vi "Tree Interaction.vi"() -> ()   [LabVIEW 2020, in "NI_VIAnCFGDataStructure.lvlib" / "Tree.lvclass"]
uses:
  <vilib>/addons/analyzer/VIAnCFGDataStructure/Tree Manager/Tree.lvclass
  <vilib>/addons/analyzer/VIAnCFGDataStructure/Tree Manager/API/Set Attribute.vi
  <vilib>/addons/analyzer/VIAnCFGDataStructure/Tree Manager/API/Get Name.vi
  <vilib>/addons/analyzer/VIAnCFGDataStructure/Tree Manager/API/Get Attribute.vi
panel:
  out "Tag":string
  out "Attribute Value":variant
  out "Clicked Attribute Name":string
  out "Clicked Tree Name":string
  in  "Stop Button":bool
  in  "Tree":string(tree)
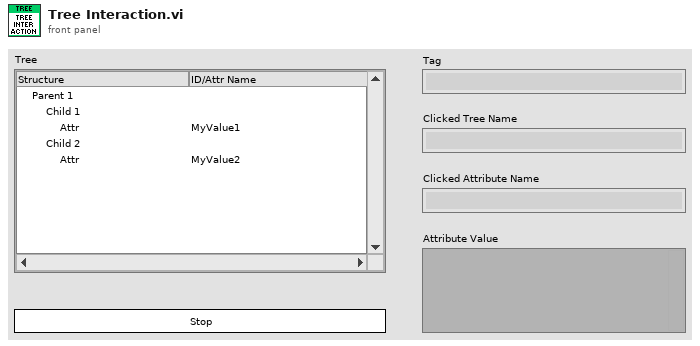
[diagram p1: front panel]
types:
  T1 = typedef "NI_VIAnCFGDataStructure.lvlib/Tree.lvclass/Session Handle.ctl" = refnum<data-value>
  T2 = typedef "LVPoint32TypeDef.ctl" = cluster{"Horizontal":i32, "Vertical":i32}
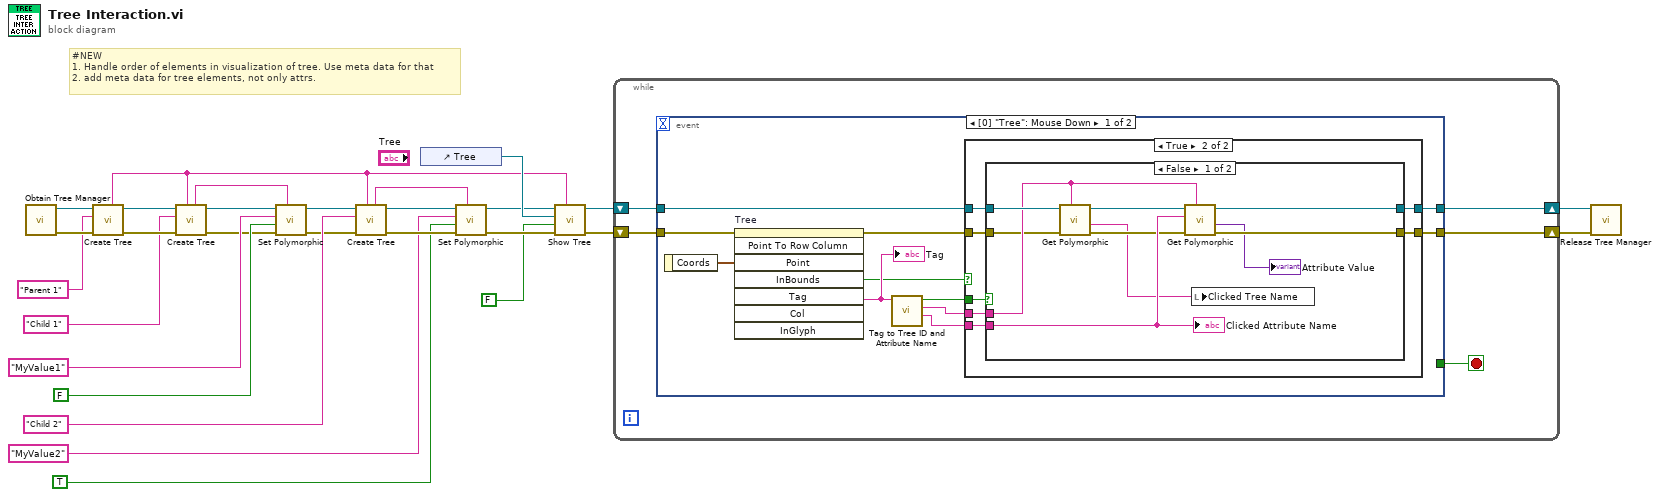
[diagram p0: block diagram]
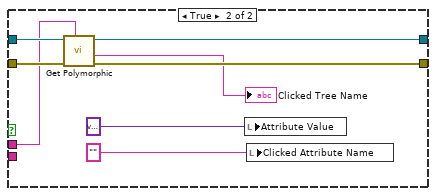
[diagram p3: hidden frame]
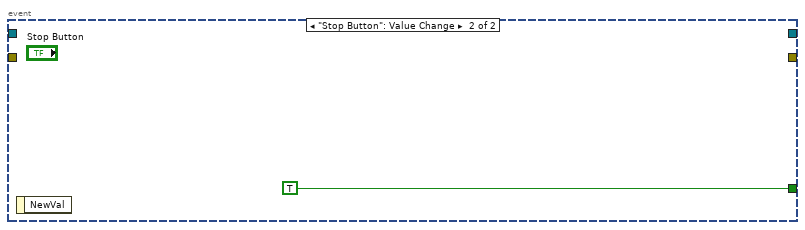
[diagram p4: hidden frame]
diagram:
  # "#NEW\n1. Handle order of elements in visualization of tree. Use meta data for that\n2. add meta data for tree elements, not only attrs."
  n1 = call <vilib>:"Obtain Tree Manager.vi"() -> ("Error Out"=w27:errorcluster, "Tree"=w28:T1)  [unwired: 10 in]
  n2 = call <vilib>:"Create Tree.vi"("Error In"=w27, "Name"="Parent 1", "Tree Manager"=w28) -> ("Error Out"=w25:errorcluster, "Tree Manager"=w26:T1, "Unique ID"=w4:string)  [unwired: 6 in]
  n3 = call <vilib>:"Create Tree.vi"("Parent ID (empty)"=w4, "Error In"=w25, "Name"="Child 1", "Tree Manager"=w26) -> ("Error Out"=w7:errorcluster, "Tree Manager"=w12:T1, "Unique ID"=w3:string)  [unwired: 5 in]
  n4 = call-poly <vilib>:"Set Polymorphic.vi"("Tree ID"=w3, "Error In"=w7, "Attribute Value"=FALSE, "Attribute Name"="MyValue1" ("Name"), "Tree Manager"=w12) -> ("Error Out"=w10:errorcluster, "Tree Manager"=w11:T1)  [unwired: 4 in, 1 out]
  n5 = call <vilib>:"Create Tree.vi"("Parent ID (empty)"=w4, "Error In"=w10, "Name"="Child 2", "Tree Manager"=w11) -> ("Error Out"=w17:errorcluster, "Tree Manager"=w18:T1, "Unique ID"=w2:string)  [unwired: 5 in]
  n6 = control-ref of="Tree"() -> (w21:refnum<vi>)
  n7 = call-poly <vilib>:"Set Polymorphic.vi"("Tree ID"=w2, "Error In"=w17, "Attribute Value"=TRUE, "Attribute Name"="MyValue2" ("Name"), "Tree Manager"=w18) -> ("Error Out"=w13:errorcluster, "Tree Manager"=w14:T1)  [unwired: 4 in, 1 out]
  n8 = call <vilib>:"Show Tree.vi"("Root ID"=w4, "Error In"=w13, "Show IDs (False)"=FALSE ("Show IDs (True)"), "Tree Ref"=w21, "Tree"=w14) -> ("Error Out"=w19:errorcluster, "Tree"=w20:T1)  [unwired: 5 in]
  n9 = while {
    shift-right: [w29] -> w6
    shift-left: w20 -> [w31]
    shift-right: [w30] -> w5
    shift-left: w19 -> [w32]
    stop <- w33 stop-if-true
    n10 = event shown="[0] \"Tree\": Mouse Down" {
      selector: _ -> [_ _]
      dyn-events: _ -> [_ _]
      timeout: _ -> [_ _]
      tunnel: [_ TRUE] -> w33
      tunnel: w32 -> [w42 _]
      tunnel: w31 -> [w38 _]
      tunnel: [w36 _] -> w30
      tunnel: [w35 _] -> w29
      event "Tree": Mouse Down {
        n11 = event-data() -> ("Coords"=w44:T2)  [unwired: 1 in]
        n12 = invoke on="Tree" class="Tree (strict)" method="Point To Row Column"(error in=w42, "Point"=w44) -> (error out=w37:errorcluster, "InBounds"=w41:bool, "Tag"=w43:string)  [unwired: 6 in, 5 out]
        "Tag" <- w43
        n13 = call <vilib>:"Tag to Tree ID and Attribute Name.vi"("Tag"=w43) -> ("Attribute Name"=w34:string, "Tree ID"=w39:string, "Tree"=w40:bool)  [unwired: 8 in]
        n14 = case shown="True" w41 {
          tunnel: w40 -> [_ w53]
          tunnel: w39 -> [_ w52]
          tunnel: w38 -> [w46 w51]
          tunnel: w37 -> [w45 w50]
          tunnel: [w45 w49] -> w36
          tunnel: [w46 w48] -> w35
          tunnel: w34 -> [_ w47]
          frame False {
          }
          frame True {
            n15 = case shown="False" w53 {
              tunnel: w52 -> [w58 w66]
              tunnel: w51 -> [w59 w71]
              tunnel: w50 -> [w55 w70]
              tunnel: [w62 w69] -> w49
              tunnel: [w63 w68] -> w48
              tunnel: w47 -> [w60 _]
              frame False {
                n16 = call-poly <vilib>:"Get Polymorphic.vi"("Tree ID"=w58, "Error In"=w55, "Tree Manager"=w59) -> ("Error Out"=w56:errorcluster, "Name"=w54:string, "Tree Manager"=w57:T1)  [unwired: 6 in]
                n17 = call-poly <vilib>:"Get Polymorphic.vi"("Tree ID"=w58, "Error In"=w56, "Attribute Name"=w60, "Tree Manager"=w57) -> ("Error Out"=w62:errorcluster, "Attribute Value"=→"Attribute Value":variant, "Tree Manager"=w63:T1)  [unwired: 4 in, 1 out]
                n18 = local write "Clicked Tree Name"(w54) -> ()
                "Clicked Attribute Name" <- w60
              }
              frame True {
                n19 = call-poly <vilib>:"Get Polymorphic.vi"("Tree ID"=w66, "Error In"=w70, "Tree Manager"=w71) -> ("Error Out"=w69:errorcluster, "Name"=→"Clicked Tree Name":string, "Tree Manager"=w68:T1)  [unwired: 6 in]
                n20 = local write "Attribute Value"(variant) -> ()
                n21 = local write "Clicked Attribute Name"("" ("Clicked Attribute Name")) -> ()
              }
            }
          }
        }
      }
      event "Stop Button": Value Change {
        n22 = event-data() -> ()  [unwired: 1 in, 1 out]
      }
    }
  }
  n23 = call <vilib>:"Release Tree Manager.vi"("Error In"=w5, "Tree"=w6) -> ()  [unwired: 9 in, 1 out]
